vi "Get COM Port Number Demo.vi"() -> (0 "COM Number":u32[](array[numeric]), 1 "Device Description":string[](array[string]))   [LabVIEW 2019]
panel:
  out "Numeric":i32
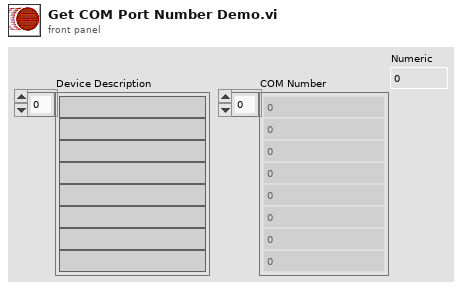
[diagram p1: front panel]
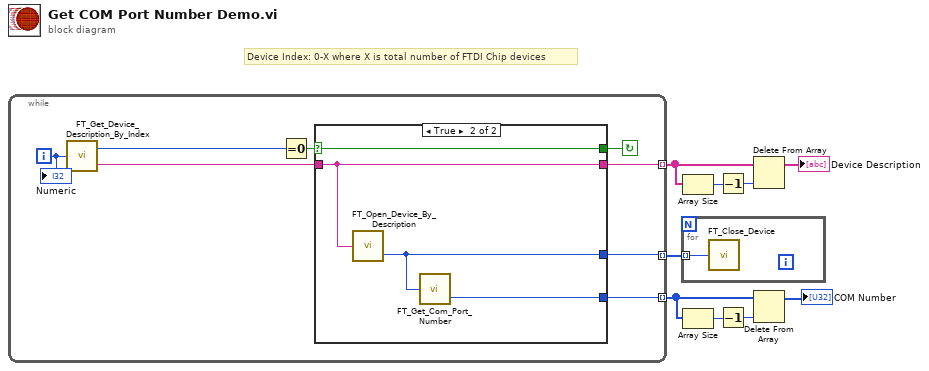
[diagram p0: block diagram]
diagram:
  # "Device Index: 0-X where X is total number of FTDI Chip devices"
  n1 = while {
    tunnel: [w13] -> w2 mode=indexing
    tunnel: [w16] -> w7 mode=indexing
    tunnel: [w10] -> w9 mode=indexing
    i -> [w17]
    stop <- w11 continue-if-true
    n2 = call "FT_Get_Device_Description_By_Index.vi"("Device Index"=w17) -> ("FT_Status"=w15:u32, "Device Description"=w14:string)
    n3 = Equal To 0?(x=w15) -> (x = 0?=w12:bool)
    n4 = case shown="True" w12 {
      selector: w12 -> [w18 w20]
      tunnel: [_ w22] -> w16
      tunnel: w14 -> [_ w21]
      tunnel: [_ w21] -> w13
      tunnel: [w18 w20] -> w11
      tunnel: [_ w19] -> w10
      frame False {
      }
      frame True {
        n5 = call "FT_Open_Device_By_Description.vi"("Device Description"=w21) -> ("Handle"=w19:u32)  [unwired: 1 out]
        n6 = call "FT_Get_Com_Port_Number.vi"("Handle"=w19) -> ("ComNumber"=w22:u32)  [unwired: 1 out]
      }
    }
    "Numeric" <- w17
  }
  n7 = for {
    tunnel: w9 -> [w23] mode=indexing
    n8 = call "FT_Close_Device.vi"("Handle"=w23) -> ()  [unwired: 1 out]
  }
  n9 = Array Size(array=w2) -> (size(s)=w4:i32)
  n10 = Array Size(array=w7) -> (size(s)=w6:i32)
  n11 = Decrement(x=w4) -> (x-1=w3:i32)
  n12 = Decrement(x=w6) -> (x-1=w5:i32)
  n13 = Delete From Array(array=w2, index=w3) -> (array with subset deleted=→"Device Description":string[])  [unwired: 1 in, 1 out]
  n14 = Delete From Array(array=w7, index=w5) -> (array with subset deleted=→"COM Number":u32[])  [unwired: 1 in, 1 out]
